vi "RVC Two Vector Transformation.vi"() -> ()   [LabVIEW 2013]
uses:
  <vilib>/robotics/Kinematics/NI_Kinematics.lvlib
panel:
  in  "Vector 2 (A)":dbl[](array[numeric])=[1.0, 0.0, 0.0]
  in  "Vector 1 (O)":dbl[](array[numeric])=[0.0, 1.0, 0.0]
  in  "Stop":bool
  out "transformation matrix":picture
  in  "Position":dbl[](array[numeric])=[1.0, 1.0, 1.0]
  out "3D Picture":refnum<vi>(3d-picture)
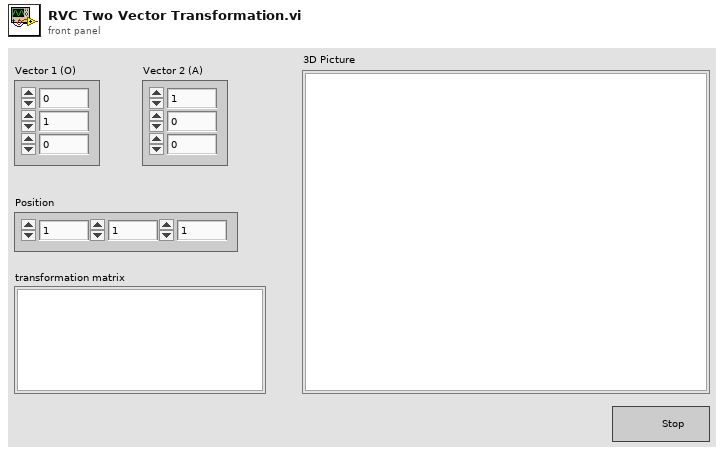
[diagram p1: front panel]
types:
  T1 = typedef "NI_Matrix.lvlib/RealMatrix.ctl" = dbl[][]
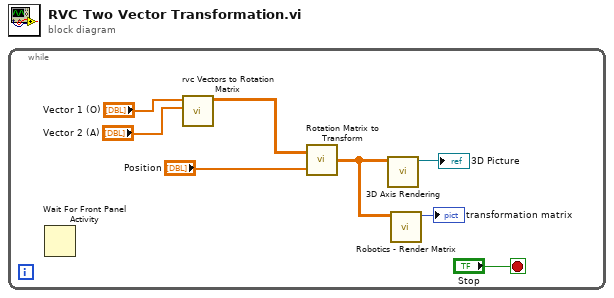
[diagram p0: block diagram]
diagram:
  n1 = while {
    stop <- "Stop" stop-if-true
    n2 = Wait For Front Panel Activity() -> ()  [unwired: 3 in, 1 out]
    n3 = call "rvc Vectors to Rotation Matrix.vi"("Vector 2 (A)"="Vector 2 (A)", "Vector 1 (O)"="Vector 1 (O)") -> ("rotation matrix"=w5:T1)  [unwired: 9 in]
    n4 = call <vilib>:"Rotation Matrix to Transform.vi"("translation vector"="Position", "rotation matrix"=w5) -> ("transform"=w3:T1)
    n5 = call "3D Axis Rendering.vi"("rotation matrix"=w3) -> ("SceneNode out"=→"3D Picture":refnum<vi>)  [unwired: 9 in, 1 out]
    n6 = call "Robotics - Render Matrix.vi"("A"=w3) -> ("picture out"=→"transformation matrix":picture)  [unwired: 10 in]
  }
